vi "read_upconfig.vi"(0 "object in":refnum<class "interface.lvclass">, 1 "段":string="应用程序交互", 2 "键数组":string[](array[string]), 3 "configuration file path":path caption="配置文件的路径", 5 "error in (no error)":errorcluster) -> (14 "object out":refnum<class "interface.lvclass">, 15 "updateconfiguration":T1={"主机"="27.154.58.30", "用户"="update", "密码"="std23506", "远程路径"="数据传输系统\\平台数据传输系统.exe", "下载文件名"="数据传输系统.exe", "软件版本"="V2.0.0.1"}, 16 "section exists?":bool caption="段存在？", 19 "error out":errorcluster)   [LabVIEW 2016, in "interface.lvclass"]
uses:
  interface.lvclass
  <vilib>/Utility/config.llb/Read Key (I32).vi
  <vilib>/Utility/config.llb/Read Key (String).vi
  <vilib>/Utility/config.llb/NI_LVConfig.lvlib
  <vilib>/Utility/Data Type/NI_Data Type.lvlib
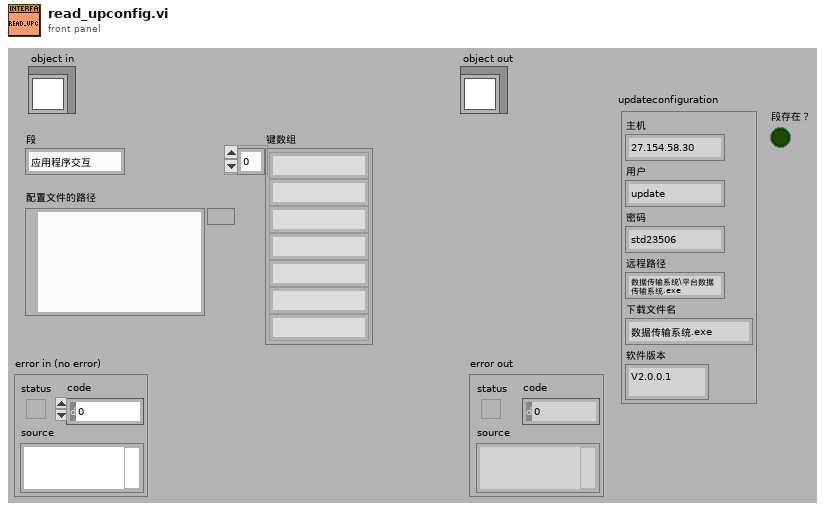
[diagram p1: front panel]
types:
  T1 = cluster{"主机":string, "用户":string, "密码":string, "远程路径":string, "下载文件名":string, "软件版本":string}
  T2 = typedef "NI_LVConfig.lvlib/Config Data RefNum.ctl" = refnum<k1>
  T3 = typedef "NI_Data Type.lvlib/Data Type.ctl" = enum8{"Invalid Type", "Void", "I8", "I16", "I32", "I64", "U8", "U16", "U32", "U64", "Single Float", "Double Float", "Extended Float", "Single Complex", "Double Complex", "Extended Complex", "Enum U8", "Enum U16", "Enum U32", "Enum U64", "Single Float With Unit", "Double Float With Unit", "Extended Float With Unit", "Single Complex with Unit", "Double Complex with Unit", "Extended Complex with Unit", "Boolean", "String", "Path", "Picture", "Tag", "Array", "Cluster", "Variant", "LV Variant", "Waveform", "Timestamp", "Digital Waveform", "Digital Data", "ExpressData", "Refnum", "External Data", "VI", "Poly VI", "LabVIEW Class Instance", "Fixed Point"}
  T4 = cluster{"[0]":string, "[1]":string, "[2]":string, "[3]":string, "[4]":string, "[5]":string}
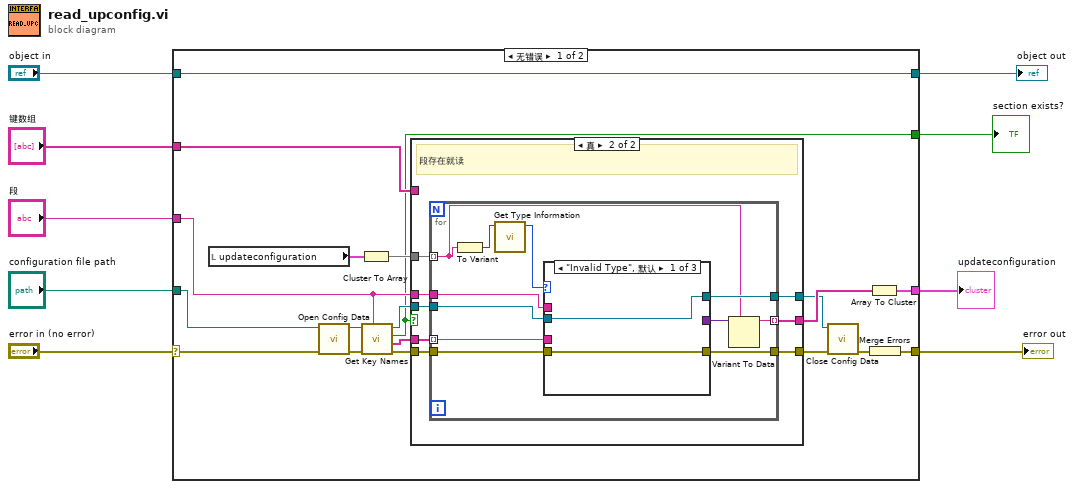
[diagram p0: block diagram]
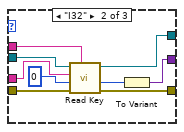
[diagram p3: hidden frame]
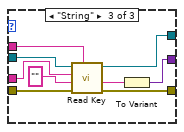
[diagram p4: hidden frame]
diagram:
  n1 = case shown="无错误" "error in (no error)" {
    selector: "error in (no error)" -> [w15 w71]
    tunnel: [w16 w71] -> w8
    tunnel: [w28 w70] -> w6
    tunnel: "object in" -> [w28 w70]
    tunnel: "configuration file path" -> [w14 _]
    tunnel: "段" -> [w13 _]
    tunnel: "键数组" -> [w12 _]
    tunnel: [w11 _] -> w2
    tunnel: [w10 _] -> w1
    frame No Error {
      n2 = local read "updateconfiguration"() -> (w25:T1)
      n3 = call <vilib>:"Open Config Data.vi"("error in (no error)"=w15, "configuration file path"=w14) -> ("error out"=w18:errorcluster, "refnum"=w17:T2)  [unwired: 7 in, 1 out]
      n4 = Cluster To Array(cluster=w25) -> (array=w26:string[])
      n5 = call <vilib>:"Get Key Names.vi"("section"=w13, "error in (no error)"=w18, "refnum"=w17) -> ("error out"=w20:errorcluster, "key names"=w21:string[], "section exists?"=w11:bool, "refnum out"=w19:T2)  [unwired: 5 in]
      n6 = case shown="真" w11 {
        tunnel: w19 -> [w30 w37]
        tunnel: w20 -> [w29 w36]
        tunnel: w21 -> [_ w38]
        tunnel: w13 -> [_ w32]
        tunnel: [_ w35] -> w27
        tunnel: [w30 w34] -> w23
        tunnel: [w29 w33] -> w24
        tunnel: w12 -> [_ _]
        tunnel: w26 -> [_ w31]
        frame False {
          # "段不存在就赋初值"
        }
        frame True {
          # "段存在就读"
          n7 = for {
            tunnel: w38 -> [w45] mode=indexing
            tunnel: w37 -> [w47]
            tunnel: w36 -> [w44]
            tunnel: w32 -> [w48]
            tunnel: [w39] -> w35 mode=indexing
            tunnel: [w46] -> w34
            tunnel: [w43] -> w33
            tunnel: w31 -> [w40] mode=indexing
            n8 = To Variant(anything=w40) -> (Variant=w42:variant)
            n9 = call <vilib>:"Get Type Information.vi"("Variant"=w42) -> ("Type"=w49:T3)  [unwired: 6 in, 4 out]
            n10 = case shown="\"Invalid Type\", 默认" w49 {
              tunnel: w48 -> [_ w59 w68]
              tunnel: w47 -> [w51 w57 w67]
              tunnel: [w51 w56 w66] -> w46
              tunnel: w45 -> [_ w58 w65]
              tunnel: w44 -> [w50 w54 w64]
              tunnel: [w50 w53 w63] -> w43
              tunnel: [_ w52 w61] -> w41
              frame "Invalid Type", Default {
              }
              frame "I32" {
                n11 = call-poly <vilib>:"Read Key.vi"("section"=w59, "error in (no error)"=w54, "default value"=0, "key"=w58, "refnum"=w57) -> ("error out"=w53:errorcluster, "value"=w55:i32, "refnum out"=w56:T2)  [unwired: 3 in, 1 out]
                n12 = To Variant(anything=w55) -> (Variant=w52:variant)
              }
              frame "String" {
                n13 = call-poly <vilib>:"Read Key.vi"("section"=w68, "error in (no error)"=w64, "default value"="", "key"=w65, "refnum"=w67) -> ("error out"=w63:errorcluster, "value"=w62:string, "refnum out"=w66:T2)  [unwired: 3 in, 1 out]
                n14 = To Variant(anything=w62) -> (Variant=w61:variant)
              }
            }
            n15 = Variant To Data(type=w40, Variant=w41) -> (data=w39:string)  [unwired: 1 in, 1 out]
          }
        }
      }
      n16 = call <vilib>:"Close Config Data.vi"("error in (no error)"=w24, "refnum"=w23) -> ("error out"=w22:errorcluster)  [unwired: 8 in, 1 out]
      n17 = Array To Cluster(array=w27) -> (cluster=w10:T4)
      n18 = Merge Errors(w22) -> (w16:errorcluster)
    }
    frame Error {
    }
  }
  "error out" <- w8
  "object out" <- w6
  "section exists?" <- w2
  "updateconfiguration" <- w1
